vi "SVT FFT Spectrum Subset (Real-Im).vi"   [LabVIEW 2017]
doc: "Computes a subset of the FFT spectrum of <B>scaled signal [EU]</B>. The subset is defined by <B>frequency range</B>. FFT results are returned as <B>real part [EU rms]</B> and <B>imaginary part [EU rms]</B>. Each block of data corresponds to a single FFT block and has to be passed individually to the this VI. You can use this polymorphic VI to analyze signals from a single channel or from N channels. The data type you wire to the <B>scaled signal [EU]</B> input determines the polymorphic instance to use."
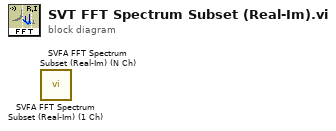
[diagram p0: block diagram]
diagram:
  n1 = call <vilib>:"SVFA FFT Spectrum Subset (Real-Im) (1 Ch).vi"() -> ()  [unwired: 13 in, 7 out]
  n2 = call <vilib>:"SVFA FFT Spectrum Subset (Real-Im) (N Ch).vi"() -> ()  [unwired: 13 in, 7 out]
